vi "Teleop.vi"(10 "Match Info":T1={"Autonomous Elapsed Seconds"=0.0, "TeleOp Elapsed Seconds"=0.0, "Disabled Elapsed Seconds"=0.0, "Visited Autonomous"=FALSE, "Visited TeleOp"=FALSE, "Visited Disabled"=FALSE, "Autonomous Settings"={"Autonomous Style"=enum."Independent", "VI Refnum"=refnum}}, 11 "Call Context":T2) -> ()   [LabVIEW 2020]
doc: "This VI is called for each TeleOp packet received from the DS where the robot is not disabled. It is often used to read from the joysticks and update I/O or to update setpoints for timed control loops. It should complete and return within 20 milliseconds or it may miss DS packets."
uses:
  <vilib>/Rock Robotics/Network Tables/NT Read Boolean.vi
  XB.vi
  RX.vi
  LX.vi
  <vilib>/Rock Robotics/Network Tables/NT Read Number.vi
  <vilib>/Rock Robotics/WPI/DriverStation/WPI_DriverStationMatch Info.ctl
  <vilib>/Rock Robotics/WPI/DriverStation/WPI_DriverStationDerivedRobotMode.ctl
panel:
  out "Sample Slider 0":dbl(slide) scale=0.0..5.0
  out "Sample Boolean 1":bool
  out "Sample Boolean 0":bool
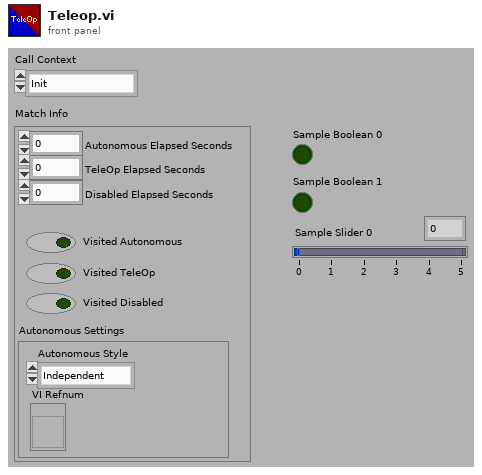
[diagram p1: front panel]
types:
  T1 = typedef "WPI_DriverStationMatch Info.ctl" = cluster{"Autonomous Elapsed Seconds":dbl, "TeleOp Elapsed Seconds":dbl, "Disabled Elapsed Seconds":dbl, "Visited Autonomous":bool, "Visited TeleOp":bool, "Visited Disabled":bool, "Autonomous Settings":cluster{"Autonomous Style":enum16{"Iterative", "Independent"}, "VI Refnum":refnum<vi>}}
  T2 = typedef "WPI_DriverStationDerivedRobotMode.ctl" = enum16{"Init", "Execute", "Stop"}
  T3 = typedef "WPI_JoystickDevRef.ctl" = cluster{"Device":T4}
  T4 = typedef "WPI_JoystickDeviceEnum.ctl" = enum16{"USB 0", "USB 1", "USB 2", "USB 3", "USB 4", "USB 5"}
  T5 = typedef "WPI_RobotDriveDevRef.ctl" = cluster{"DevStatus":errorcluster, "Motors[]":T6[], "Square Inputs":bool, "Max Output":dbl}
  T6 = typedef "WPI_MotorControlDeviceRef.ctl" = cluster{"DeviceStatus":errorcluster, "Type":T7, "PWM":cluster{"PWM Channel":T8, "DeadBand":T9}, "CAN":cluster{"Device Number":u8, "SetOutput VI Ref":variant, "GetOutput VI Ref":variant, "Enable VI Ref":variant, "Disable VI Ref":variant, "Data":variant}, "Invert":bool, "DIO PWM":cluster{"PWM \"Enable\" Channel":T8, "DIOChannel":T10, "PWM Rate":dbl}}
  T7 = typedef "WPI_MotorControlType.ctl" = enum16{"PWM", "CAN", "DIO PWM"}
  T8 = typedef "FPGA_DIOPWMChannel.ctl" = enum8{"PWM 0", "PWM 1", "PWM 2", "PWM 3", "PWM 4", "PWM 5", "PWM 6", "PWM 7", "PWM 8", "PWM 9", "PWM MXP 0", "PWM MXP 1", "PWM MXP 2", "PWM MXP 3", "PWM MXP 4", "PWM MXP 5", "PWM MXP 6", "PWM MXP 7", "PWM MXP 8", "PWM MXP 9", "Invalid"}
  T9 = typedef "WPI_PWMDeadband.ctl" = cluster{"Name":string, "maxPositivePwm":i32, "minPositivePwm":i32, "centerPwm":i32, "maxNegativePwm":i32, "minNegativePwm":i32, "angularRange":u16}
  T10 = typedef "FPGA_DIOChannel.ctl" = enum8{"DIO 0", "DIO 1", "DIO 2", "DIO 3", "DIO 4", "DIO 5", "DIO 6", "DIO 7", "DIO 8", "DIO 9", "DIO MXP 0", "DIO MXP 1", "DIO MXP 2", "DIO MXP 3", "DIO MXP 4", "DIO MXP 5", "DIO MXP 6", "DIO MXP 7", "DIO MXP 8", "DIO MXP 9", "DIO MXP 10", "DIO MXP 11", "DIO MXP 12", "DIO MXP 13", "DIO MXP 14", "DIO MXP 15", "SPI Port CS1", "SPI Port CS2", "SPI Port CS3", "SPI Port MISO", "SPI Port MOSI", "Invalid"}
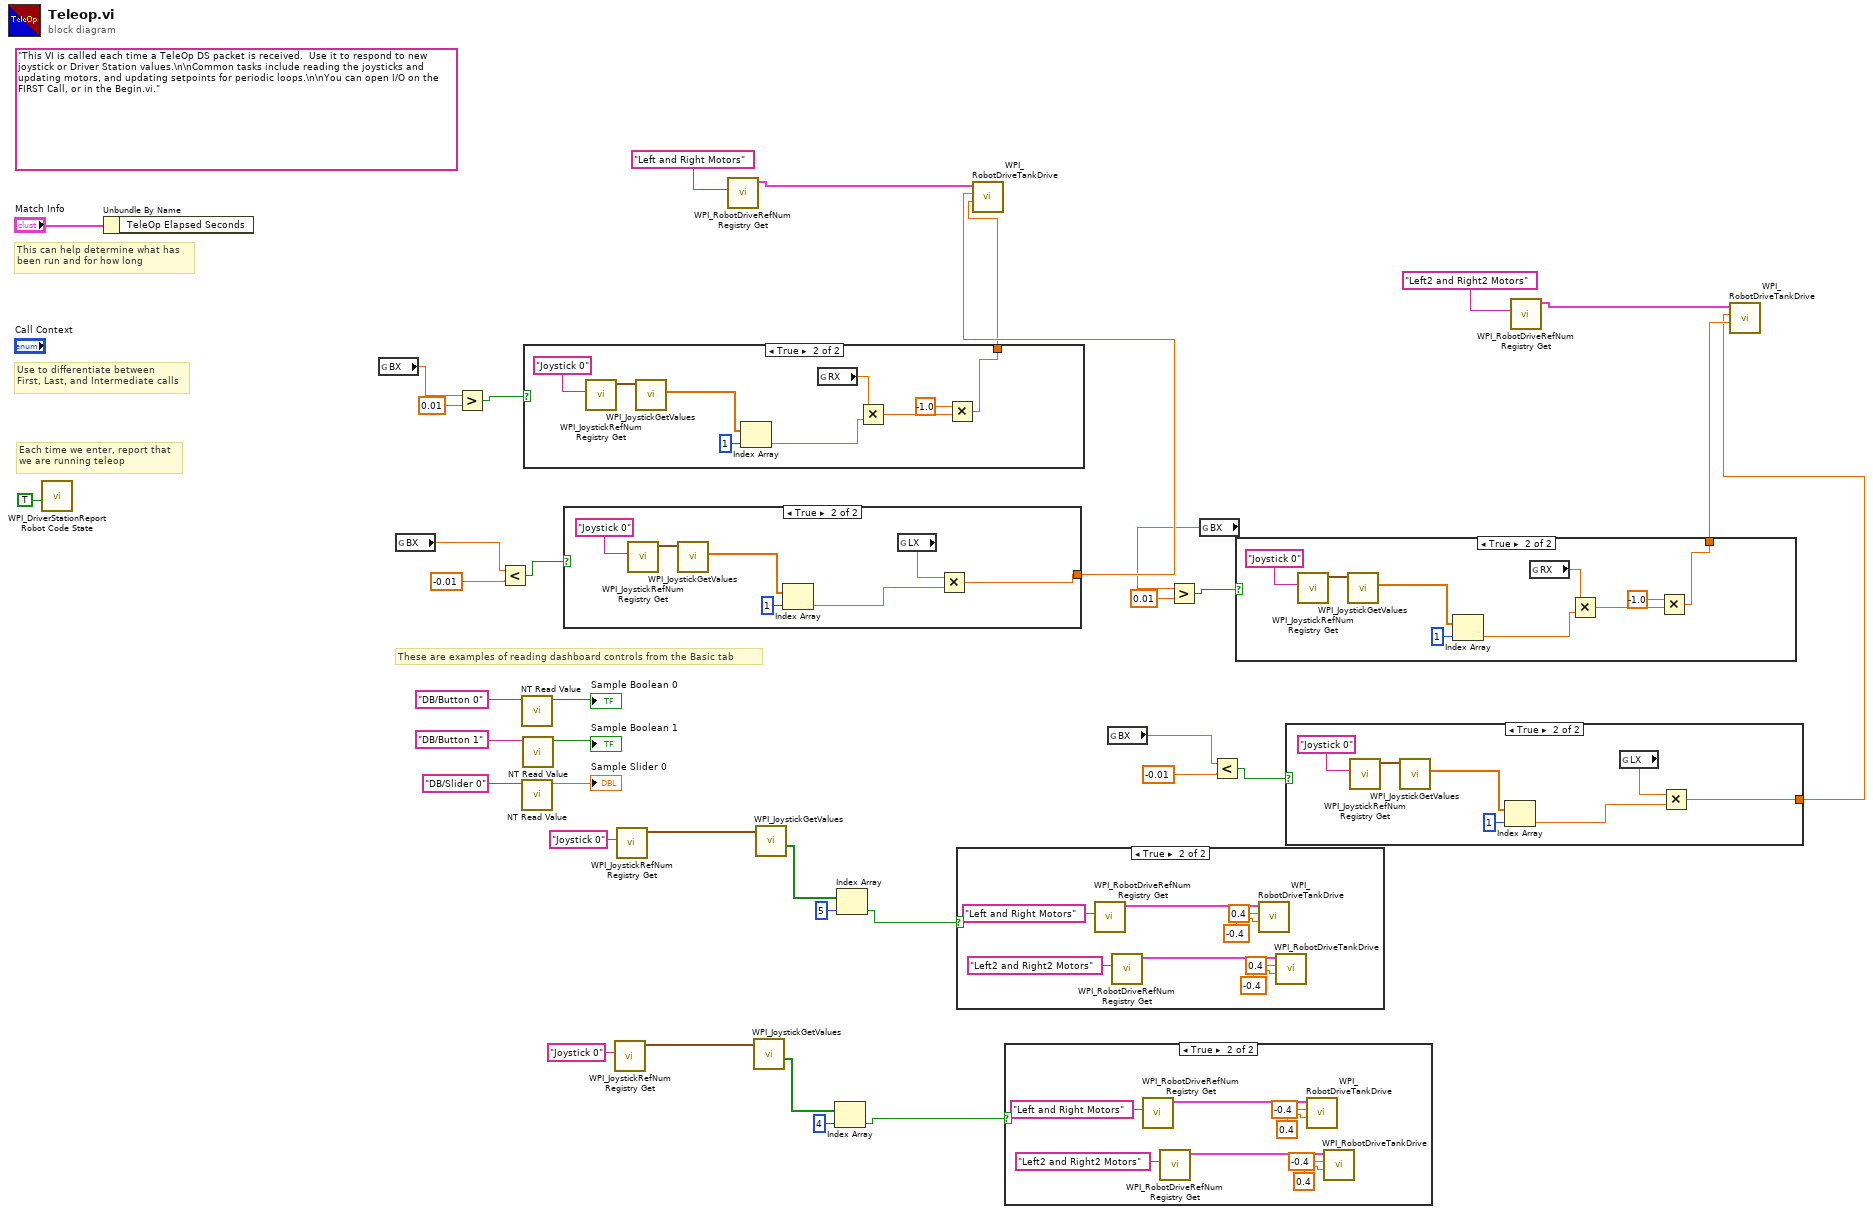
[diagram p0: block diagram]
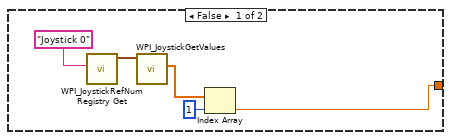
[diagram p4: hidden frame]
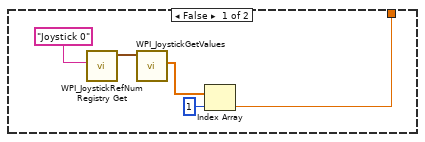
[diagram p5: hidden frame]
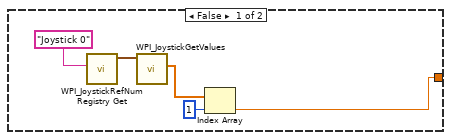
[diagram p6: hidden frame]
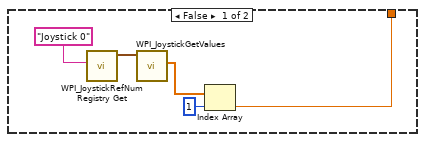
[diagram p7: hidden frame]
diagram:
  (unwired) "This VI is called each time a TeleOp DS packet is received.  Use it to respond to new joystick or Driver Station values.\n\nCommon tasks include reading the joysticks and updating motors, and updating setpoints for periodic loops.\n\nYou can open I/O on the FIRST Call, or in the Begin.vi."
  # "These are examples of reading dashboard controls from the Basic tab"
  # "Each time we enter, report that\nwe are running teleop"
  # "Use to differentiate between\nFirst, Last, and Intermediate calls"
  # "This can help determine what has\nbeen run and for how long"
  n1 = call <vilib>:"WPI_DriverStationReport Robot Code State.vi"("TeleOp"=TRUE ("Autonomous")) -> ()  [unwired: 10 in, 1 out]
  n2 = Unbundle By Name("Match Info") -> ()  [unwired: 1 out]
  n3 = global read "XB.vi" "BX"() -> (w28:dbl)
  n4 = global read "XB.vi" "BX"() -> (w25:dbl)
  n5 = Greater?(x=w28, y=0.01) -> (0:w26:bool)
  n6 = Less?(x=w25, y=-0.01) -> (x < y?=w23:bool)
  n7 = call-poly <vilib>:"NT Read Value.vi"("Name"="DB/Button 0" ("refnum name")) -> ("Boolean"=→"Sample Boolean 0":bool)  [unwired: 9 in, 1 out]
  n8 = call-poly <vilib>:"NT Read Value.vi"("Name"="DB/Slider 0" ("refnum name")) -> ("Numeric"=→"Sample Slider 0":dbl)  [unwired: 9 in, 1 out]
  n9 = call-poly <vilib>:"NT Read Value.vi"("Name"="DB/Button 1" ("refnum name")) -> ("Boolean"=→"Sample Boolean 1":bool)  [unwired: 9 in, 1 out]
  n10 = case shown="True" w26 {
    tunnel: [w39 w44] -> w19
    frame False {
      n11 = call <vilib>:"WPI_JoystickRefNum Registry Get.vi"("refnum name"="Joystick 0") -> ("JoystickDevRef"=w42:T3)  [unwired: 1 in, 9 out]
      n12 = call <vilib>:"WPI_JoystickGetValues.vi"("JoystickDevRef"=w42) -> ("Axes"=w43:dbl[])  [unwired: 6 in, 4 out]
      n13 = Index Array(array=w43, index=1) -> (element=w39:dbl)
    }
    frame True {
      n14 = call <vilib>:"WPI_JoystickRefNum Registry Get.vi"("refnum name"="Joystick 0") -> ("JoystickDevRef"=w50:T3)  [unwired: 1 in, 9 out]
      n15 = call <vilib>:"WPI_JoystickGetValues.vi"("JoystickDevRef"=w50) -> ("Axes"=w48:dbl[])  [unwired: 6 in, 4 out]
      n16 = Index Array(array=w48, index=1) -> (element=w47:dbl)
      n17 = global read "RX.vi" "RX"() -> (w51:dbl)
      n18 = Multiply(x=w51, y=w47) -> (x*y=w46:dbl)
      n19 = Multiply(x=-1.0, y=w46) -> (x*y=w44:dbl)
    }
  }
  n20 = case shown="True" w23 {
    tunnel: [w53 w58] -> w20
    frame False {
      n21 = call <vilib>:"WPI_JoystickRefNum Registry Get.vi"("refnum name"="Joystick 0") -> ("JoystickDevRef"=w56:T3)  [unwired: 1 in, 9 out]
      n22 = call <vilib>:"WPI_JoystickGetValues.vi"("JoystickDevRef"=w56) -> ("Axes"=w57:dbl[])  [unwired: 6 in, 4 out]
      n23 = Index Array(array=w57, index=1) -> (element=w53:dbl)
    }
    frame True {
      n24 = call <vilib>:"WPI_JoystickRefNum Registry Get.vi"("refnum name"="Joystick 0") -> ("JoystickDevRef"=w63:T3)  [unwired: 1 in, 9 out]
      n25 = call <vilib>:"WPI_JoystickGetValues.vi"("JoystickDevRef"=w63) -> ("Axes"=w61:dbl[])  [unwired: 6 in, 4 out]
      n26 = Index Array(array=w61, index=1) -> (element=w59:dbl)
      n27 = global read "LX.vi" "LX"() -> (w60:dbl)
      n28 = Multiply(x=w60, y=w59) -> (x*y=w58:dbl)
    }
  }
  n29 = call <vilib>:"WPI_JoystickRefNum Registry Get.vi"("refnum name"="Joystick 0") -> ("JoystickDevRef"=w9:T3)  [unwired: 9 in, 1 out]
  n30 = call <vilib>:"WPI_JoystickRefNum Registry Get.vi"("refnum name"="Joystick 0") -> ("JoystickDevRef"=w5:T3)  [unwired: 9 in, 1 out]
  n31 = call <vilib>:"WPI_RobotDriveRefNum Registry Get.vi"("refnum name"="Left and Right Motors") -> ("RobotDriveDevRef"=w29:T5)  [unwired: 1 in, 9 out]
  n32 = call <vilib>:"WPI_JoystickGetValues.vi"("JoystickDevRef"=w9) -> ("Buttons"=w8:bool[])  [unwired: 6 in, 4 out]
  n33 = call <vilib>:"WPI_JoystickGetValues.vi"("JoystickDevRef"=w5) -> ("Buttons"=w4:bool[])  [unwired: 6 in, 4 out]
  n34 = Index Array(array=w8, index=4) -> (element=w1:bool)
  n35 = Index Array(array=w4, index=5) -> (element=w2:bool)
  n36 = case shown="True" w2 {
    frame False {
    }
    frame True {
      n37 = call <vilib>:"WPI_RobotDriveRefNum Registry Get.vi"("refnum name"="Left and Right Motors") -> ("RobotDriveDevRef"=w72:T5)  [unwired: 9 in, 1 out]
      n38 = call <vilib>:"WPI_RobotDriveRefNum Registry Get.vi"("refnum name"="Left2 and Right2 Motors") -> ("RobotDriveDevRef"=w71:T5)  [unwired: 9 in, 1 out]
      n39 = call <vilib>:"WPI_RobotDriveTankDrive.vi"("Right axis value"=-0.4, "Left axis value"=0.4, "RobotDriveDevRef"=w72) -> ()  [unwired: 6 in, 3 out]
      n40 = call <vilib>:"WPI_RobotDriveTankDrive.vi"("Right axis value"=-0.4, "Left axis value"=0.4, "RobotDriveDevRef"=w71) -> ()  [unwired: 6 in, 3 out]
    }
  }
  n41 = call <vilib>:"WPI_RobotDriveTankDrive.vi"("Right axis value"=w19, "Left axis value"=w20, "RobotDriveDevRef"=w29) -> ()  [unwired: 6 in, 3 out]
  n42 = case shown="True" w1 {
    frame False {
    }
    frame True {
      n43 = call <vilib>:"WPI_RobotDriveRefNum Registry Get.vi"("refnum name"="Left and Right Motors") -> ("RobotDriveDevRef"=w80:T5)  [unwired: 9 in, 1 out]
      n44 = call <vilib>:"WPI_RobotDriveRefNum Registry Get.vi"("refnum name"="Left2 and Right2 Motors") -> ("RobotDriveDevRef"=w79:T5)  [unwired: 9 in, 1 out]
      n45 = call <vilib>:"WPI_RobotDriveTankDrive.vi"("Right axis value"=0.4, "Left axis value"=-0.4, "RobotDriveDevRef"=w80) -> ()  [unwired: 6 in, 3 out]
      n46 = call <vilib>:"WPI_RobotDriveTankDrive.vi"("Right axis value"=0.4, "Left axis value"=-0.4, "RobotDriveDevRef"=w79) -> ()  [unwired: 6 in, 3 out]
    }
  }
  n47 = global read "XB.vi" "BX"() -> (w15:dbl)
  n48 = global read "XB.vi" "BX"() -> (w18:dbl)
  n49 = Greater?(x=w18, y=0.01) -> (0:w16:bool)
  n50 = Less?(x=w15, y=-0.01) -> (x < y?=w13:bool)
  n51 = case shown="True" w16 {
    tunnel: [w81 w86] -> w12
    frame False {
      n52 = call <vilib>:"WPI_JoystickRefNum Registry Get.vi"("refnum name"="Joystick 0") -> ("JoystickDevRef"=w84:T3)  [unwired: 1 in, 9 out]
      n53 = call <vilib>:"WPI_JoystickGetValues.vi"("JoystickDevRef"=w84) -> ("Axes"=w85:dbl[])  [unwired: 6 in, 4 out]
      n54 = Index Array(array=w85, index=1) -> (element=w81:dbl)
    }
    frame True {
      n55 = call <vilib>:"WPI_JoystickRefNum Registry Get.vi"("refnum name"="Joystick 0") -> ("JoystickDevRef"=w92:T3)  [unwired: 1 in, 9 out]
      n56 = call <vilib>:"WPI_JoystickGetValues.vi"("JoystickDevRef"=w92) -> ("Axes"=w90:dbl[])  [unwired: 6 in, 4 out]
      n57 = Index Array(array=w90, index=1) -> (element=w89:dbl)
      n58 = global read "RX.vi" "RX"() -> (w93:dbl)
      n59 = Multiply(x=w93, y=w89) -> (x*y=w88:dbl)
      n60 = Multiply(x=-1.0, y=w88) -> (x*y=w86:dbl)
    }
  }
  n61 = case shown="True" w13 {
    tunnel: [w95 w100] -> w11
    frame False {
      n62 = call <vilib>:"WPI_JoystickRefNum Registry Get.vi"("refnum name"="Joystick 0") -> ("JoystickDevRef"=w98:T3)  [unwired: 1 in, 9 out]
      n63 = call <vilib>:"WPI_JoystickGetValues.vi"("JoystickDevRef"=w98) -> ("Axes"=w99:dbl[])  [unwired: 6 in, 4 out]
      n64 = Index Array(array=w99, index=1) -> (element=w95:dbl)
    }
    frame True {
      n65 = call <vilib>:"WPI_JoystickRefNum Registry Get.vi"("refnum name"="Joystick 0") -> ("JoystickDevRef"=w105:T3)  [unwired: 1 in, 9 out]
      n66 = call <vilib>:"WPI_JoystickGetValues.vi"("JoystickDevRef"=w105) -> ("Axes"=w103:dbl[])  [unwired: 6 in, 4 out]
      n67 = Index Array(array=w103, index=1) -> (element=w101:dbl)
      n68 = global read "LX.vi" "LX"() -> (w102:dbl)
      n69 = Multiply(x=w102, y=w101) -> (x*y=w100:dbl)
    }
  }
  n70 = call <vilib>:"WPI_RobotDriveRefNum Registry Get.vi"("refnum name"="Left2 and Right2 Motors") -> ("RobotDriveDevRef"=w21:T5)  [unwired: 1 in, 9 out]
  n71 = call <vilib>:"WPI_RobotDriveTankDrive.vi"("Right axis value"=w12, "Left axis value"=w11, "RobotDriveDevRef"=w21) -> ()  [unwired: 6 in, 3 out]
